vi "A-Lockin_Vsg-JKISM.vi"(8 "error in (no error)":errorcluster, 11 "SweepControl":refnum<class "SweepControl.lvclass">) -> (0 "error out":errorcluster)   [LabVIEW 2016, in "Transport.lvclass"]
uses:
  <userlib>/LevyLab/Transport/Transport/Transport.lvclass
  <userlib>/LevyLab/Lockin-Multichannel/Typedefs/AO-cluster.ctl
  <userlib>/LevyLab/Lockin-Multichannel/Typedefs/AO_Amp-array.ctl
  <userlib>/LevyLab/Lockin-Multichannel/Typedefs/AO_DC-array.ctl
  <userlib>/LevyLab/Lockin-Multichannel/Typedefs/AO_f-array.ctl
  <userlib>/LevyLab/Lockin-Multichannel/Typedefs/AO_phi-array.ctl
  <userlib>/LevyLab/Lockin-Multichannel/Typedefs/Function-array.ctl
  <userlib>/LevyLab/Lockin-Multichannel/Typedefs/Function-enum.ctl
  <userlib>/LevyLab/Transport/SweepControl/SweepControl.lvclass
  <userlib>/LevyLab/Transport/SweepControl/Typedefs/Cluster - ScanParamters.ctl
  <userlib>/LevyLab/Levylab Instruments/Instrument Types/Cryostat/Instrument.Cryostat.lvclass
  <userlib>/LevyLab/LV to ITX/LVtoITX.lvclass
  <userlib>/LevyLab/Transport/Control Experiment/Control Experiment.lvclass
panel:
  in  "OK":bool
  in  "Tab Control":enum32{"lockin/SG Control", "Data", "Other"}(tab)
  in  "Channels: AO":T1={"AO amp (V)"=[0.0002, 0.0, 0.0, 0.0, 0.0, 0.0, 0.0, 0.0], "AO DC (V)"=[0.00025, 0.0, 0.0, 0.0, 0.0, 0.0, 0.0, 0.0], "AO f (Hz)"=[13.0, 13.0, 13.0, 13.0, 13.0, 13.0, 13.0, 13.0], "AO phi (°)"=[0.0, 0.0, 0.0, 0.0, 0.0, 0.0, 0.0, 0.0], "function"=[enum."Sine", enum."Sine", enum."Sine", enum."Sine", enum."Sine", enum."Sine", enum."Sine", enum."Sine"], "I+"=[]} {"AO f (Hz)" min=0.001 max=10000.0; "AO DC (V)" format="%.3p"; "AO amp (V)" format="%.3p"}
  in  "Vmax (end)":dbl=1.0 format="%#_3p"
  in  "Vmin (start)":dbl format="%#_3p"
  in  "dV":dbl=0.1 format="%#_3p"
  in  "Experiment Description":string="write a description of THIS experiment here"
  in  "Experiment Folder":string="folder name"
  in  "wait after setting Vsg (ms)":u32
  in  "Initial wait (ms)":u32=100
  in  "side gate channel":i32=1 min=1
  in  "Physical Channel":tag="Dev2/ao0" caption="Back Gate Channel"
  in  "Sweep":enum16{"Vsg", "Vbg"}(ring)
  in  "cycles (1,2,...)":i32=1 min=1 step=1
  in  "phase":dbl
  in  "function (ramp)":enum16{"Ramp", "Triangle", "Sine"}(ring)
  in  "set parameter to initial value?":bool
  out "G 4T":cluster{"Y":dbl[], "Y":dbl[]}[](graph)
  out "Lockins":cluster{"Y":dbl[], "Y":dbl[]}[](graph)
  out "Lockins 2":cluster{"Y":dbl[], "Y":dbl[]}[](graph)
  # "1"
  # "2"
  # "3"
  # "4"
  # "5"
  # "6"
  # "7"
  # "8"
  # "dynamically name the traces"
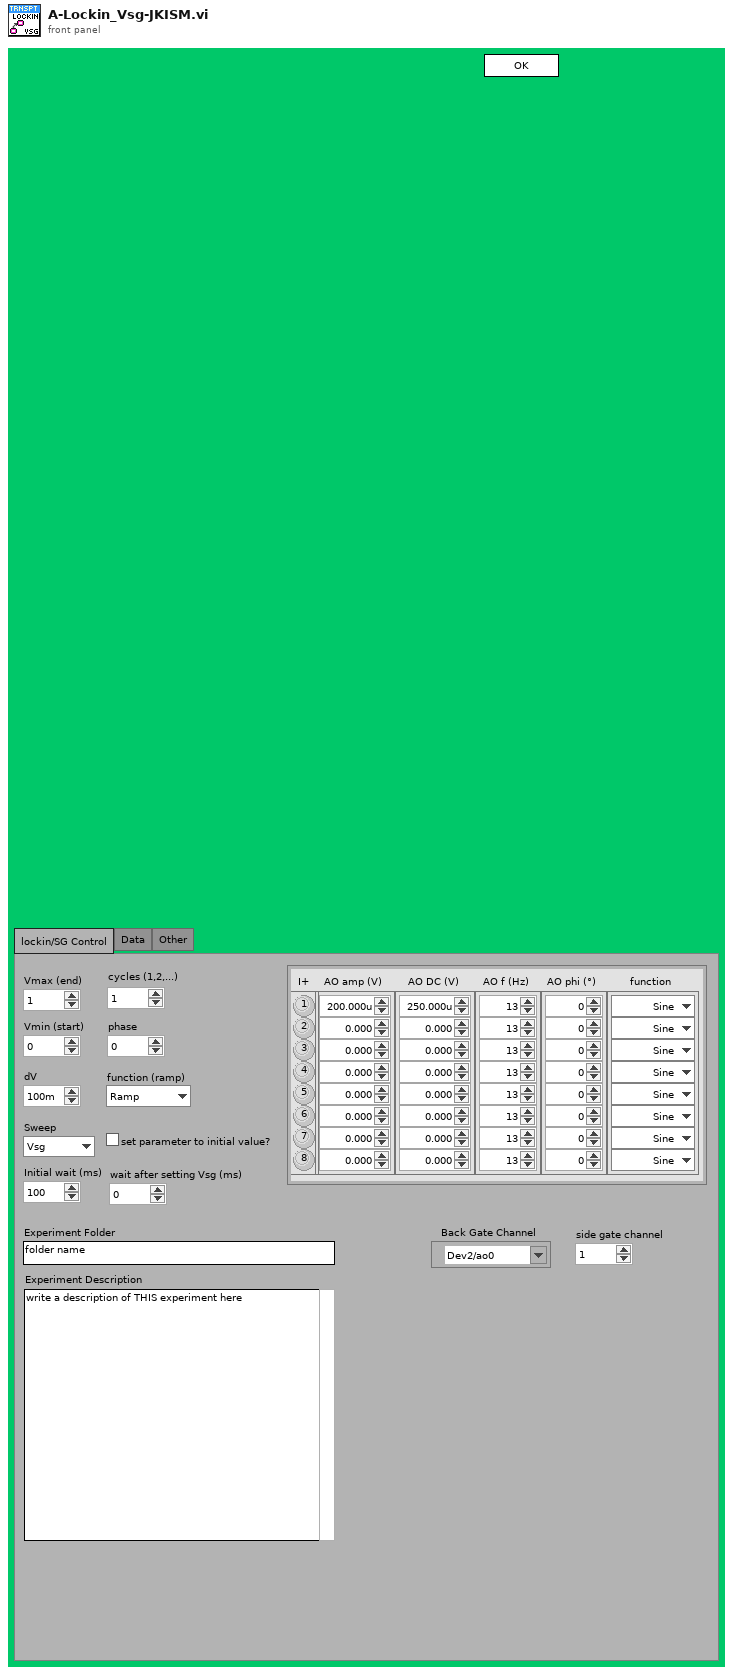
[diagram p1: front panel]
types:
  T1 = typedef "AO-cluster.ctl" = cluster{"AO amp (V)":T2, "AO DC (V)":T3, "AO f (Hz)":T4, "AO phi (°)":T5, "function":T6, "I+":bool[]}
  T2 = typedef "AO_Amp-array.ctl" = dbl[]
  T3 = typedef "AO_DC-array.ctl" = dbl[]
  T4 = typedef "AO_f-array.ctl" = dbl[]
  T5 = typedef "AO_phi-array.ctl" = dbl[]
  T6 = typedef "Function-array.ctl" = T7[]
  T7 = typedef "Function-enum.ctl" = enum16{"Sine", "Triangle", "Square", "Sawtooth"}
  T8 = enum32{"Bad", "Idle", "Run top level", "Running"}
  T9 = enum32{"invalid app kind", "Development System", "Run Time System", "Student Edition", "Embedded LabVIEW", "Evaluation", "Custom"}
  T10 = enum32{"Invalid", "Standard", "Closed", "Hidden", "Minimized", "Maximized"}
  T11 = typedef "SweepControl.lvclass/Cluster - ScanParamters.ctl" = cluster{"Start":dbl, "End":dbl, "Step":dbl, "Rate":dbl, "wait (ms)":u32, "Address":string, "Channel":i32}
  T12 = cluster{"Core":cluster{"Current VI Reference":refnum<vi>, "Close Panel on Exit?":bool}, "top level?":bool, "SweepControl":refnum<class "SweepControl.lvclass">, "Instrument":cluster{"Temperature":refnum<class "Instrument.Cryostat.lvclass">, "Magnet":refnum<class "Instrument.Cryostat.lvclass">, "Rotator":refnum<class "Instrument.Cryostat.lvclass">, "Level":refnum<class "Instrument.Cryostat.lvclass">}, "file":cluster{"path":path, "Experiment Folder":string, "device":string, "Comments":string}, "data":cluster{"Result X":dbl[], "Result Y":dbl[], "Data":cluster{"Y  Array":dbl[]}[], "wavenames":string[], "All Result X":dbl[][], "All Result Y":dbl[][]}, "lockin address":string, "Channels: AO":T1, "Temperature (K)":dbl, "Field (T)":dbl, "ramp rate (T/min)":dbl, "inner scan":T11, "All Parameters":dbl[], "loop index":i32, "Current Parameter":dbl}
  T13 = cluster{"Temperature":refnum<class "Instrument.Cryostat.lvclass">, "Magnet":refnum<class "Instrument.Cryostat.lvclass">, "Rotator":refnum<class "Instrument.Cryostat.lvclass">, "Level":refnum<class "Instrument.Cryostat.lvclass">}
  T14 = cluster{"Result X":dbl[], "Result Y":dbl[], "Data":cluster{"Y  Array":dbl[]}[], "wavenames":string[], "All Result X":dbl[][], "All Result Y":dbl[][]}
  T15 = cluster{"path":path, "Experiment Folder":string, "device":string, "Comments":string}
  T16 = cluster{"Current VI Reference":refnum<vi>, "Close Panel on Exit?":bool}
  T17 = typedef "SweepControl.lvclass/ScanParamters.ctl" = T11[]
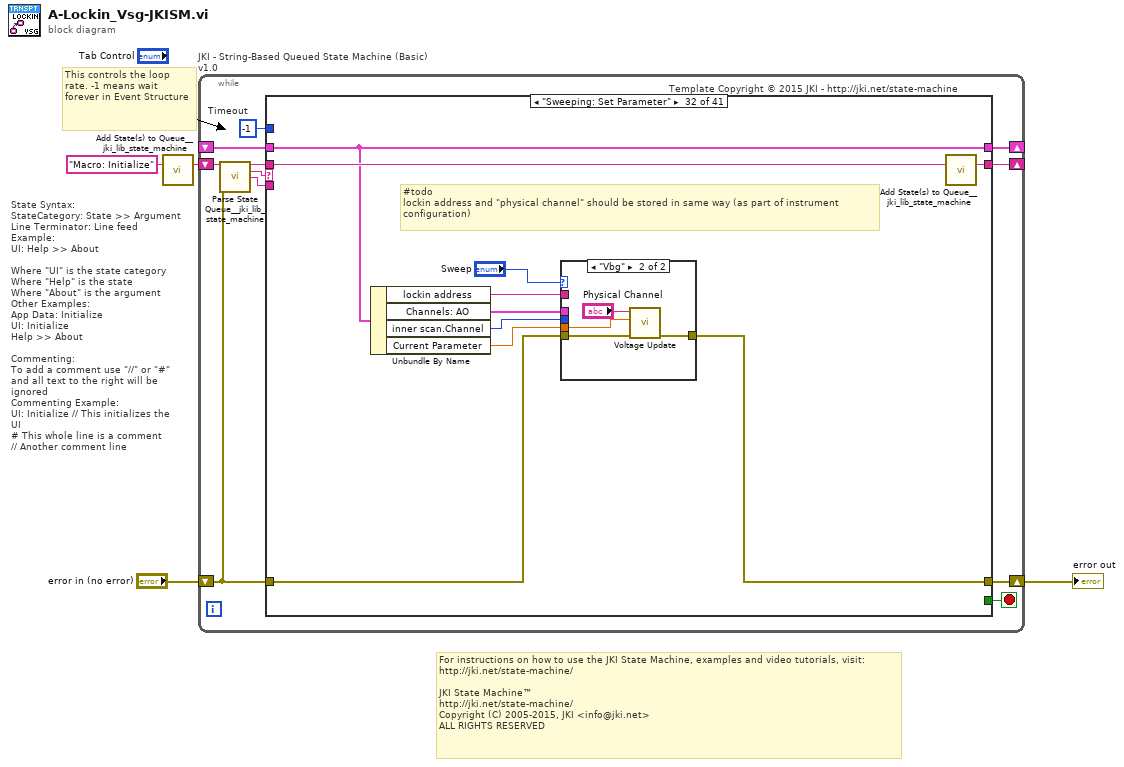
[diagram p0: block diagram]
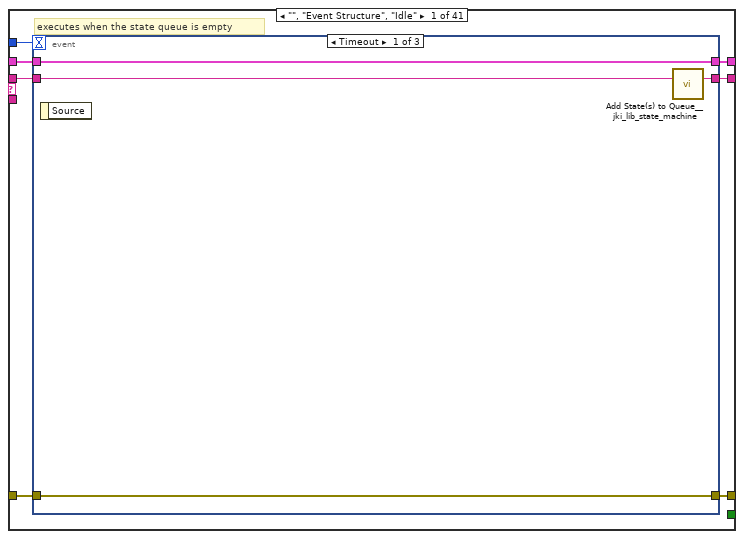
[diagram p2: hidden frame]
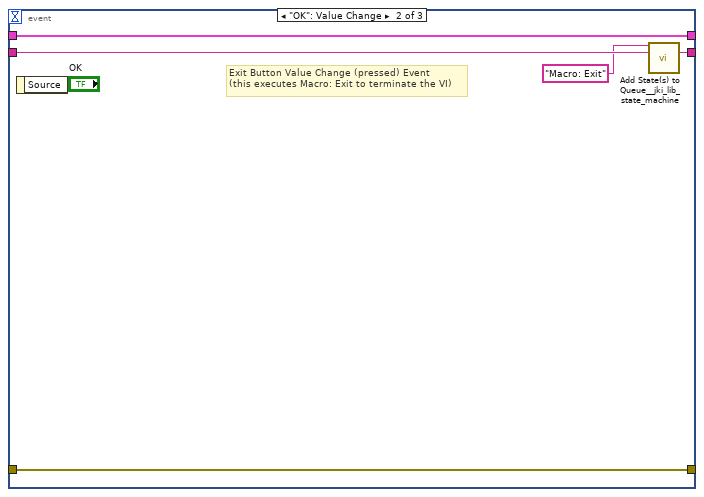
[diagram p3: hidden frame]
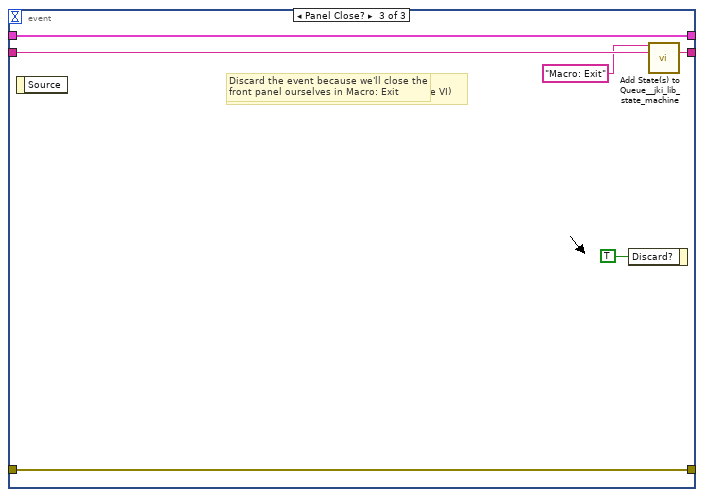
[diagram p4: hidden frame]
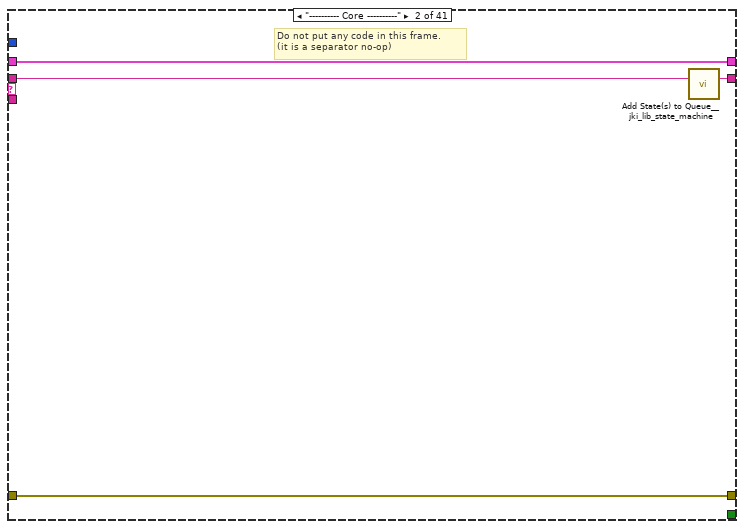
[diagram p5: hidden frame]
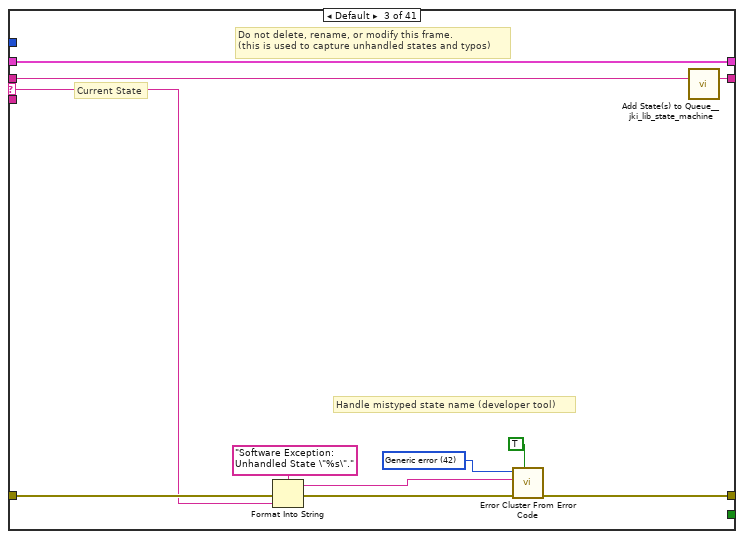
[diagram p6: hidden frame]
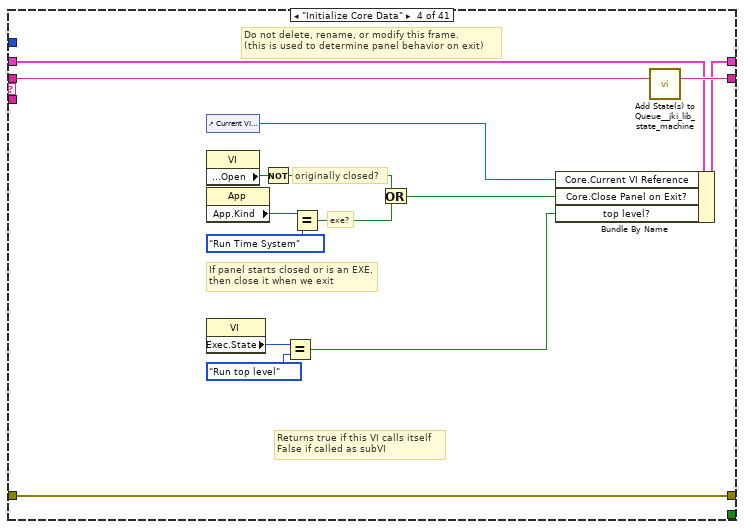
[diagram p7: hidden frame]
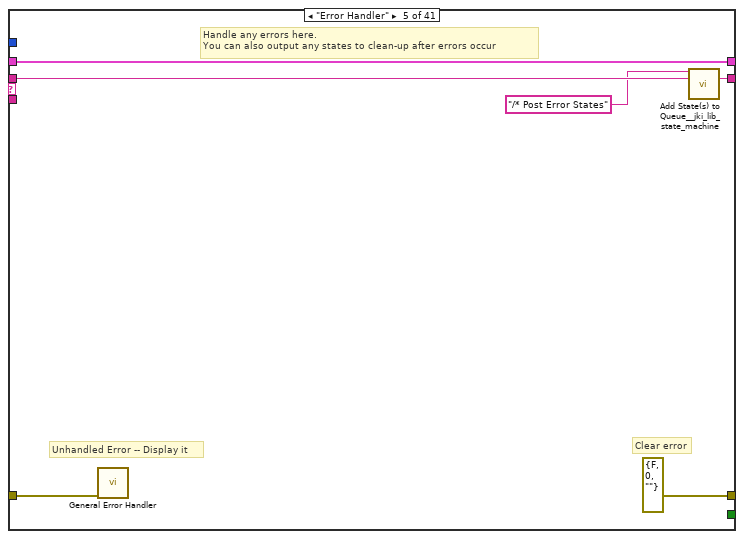
[diagram p8: hidden frame]
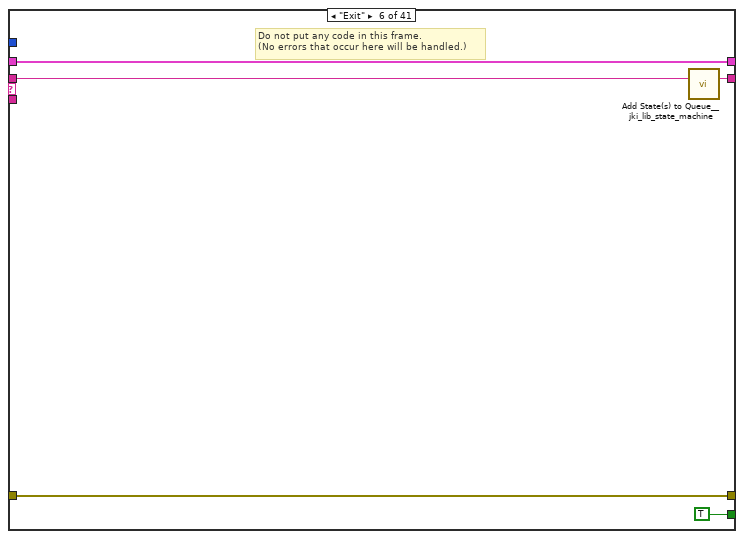
[diagram p9: hidden frame]
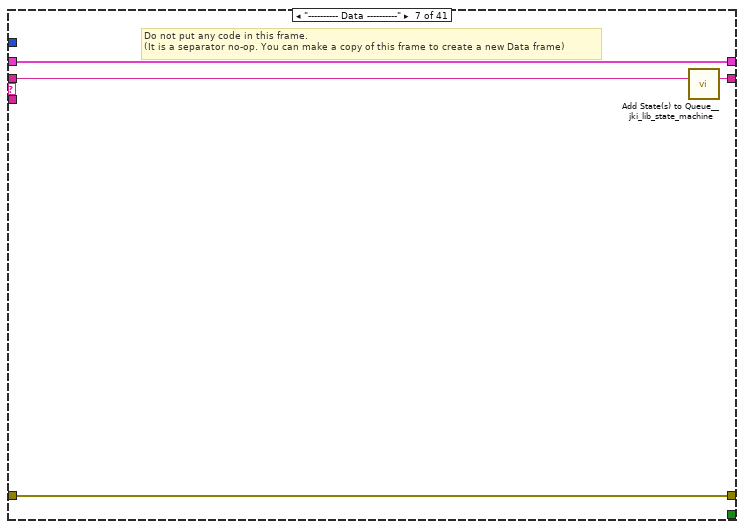
[diagram p10: hidden frame]
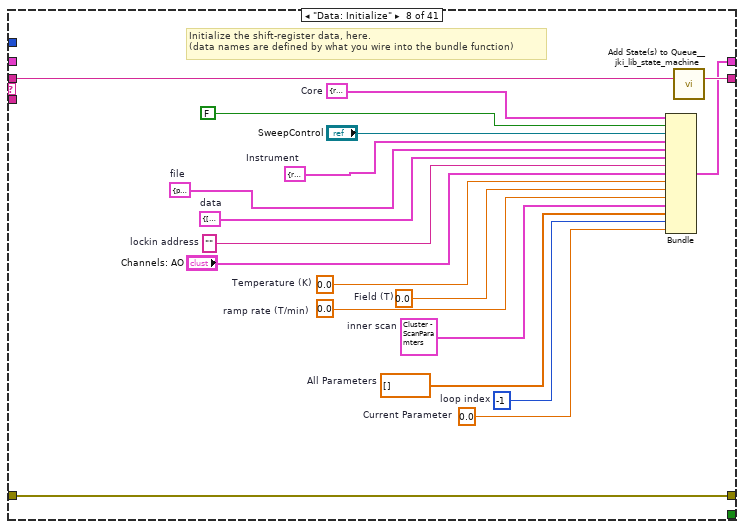
[diagram p11: hidden frame]
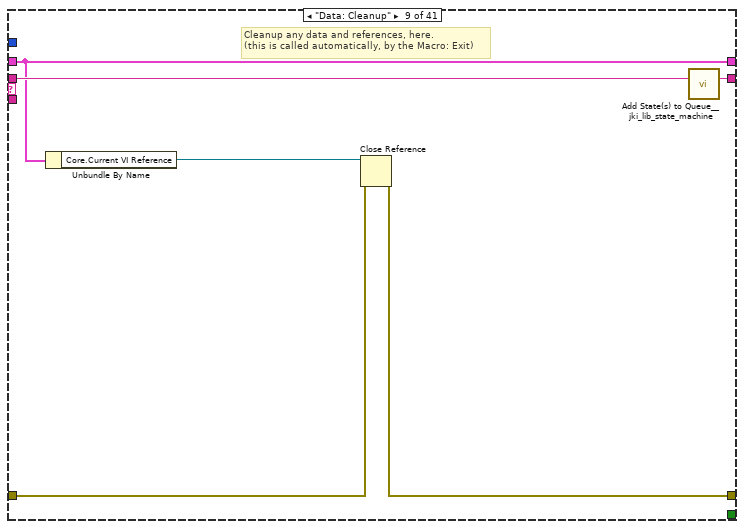
[diagram p12: hidden frame]
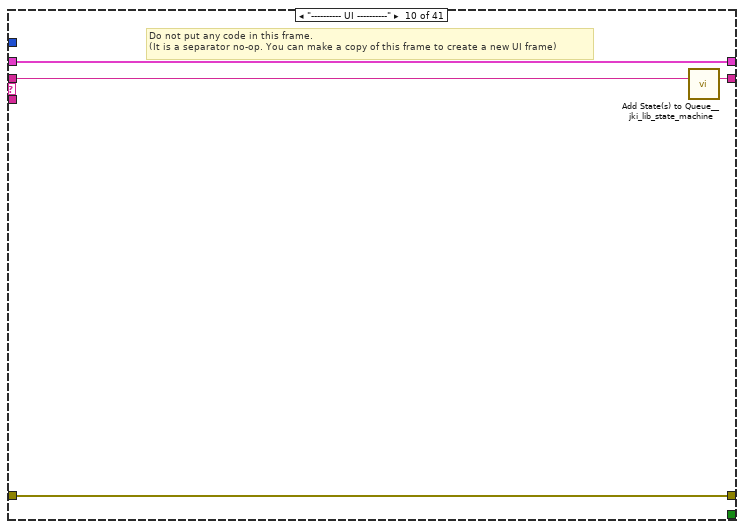
[diagram p13: hidden frame]
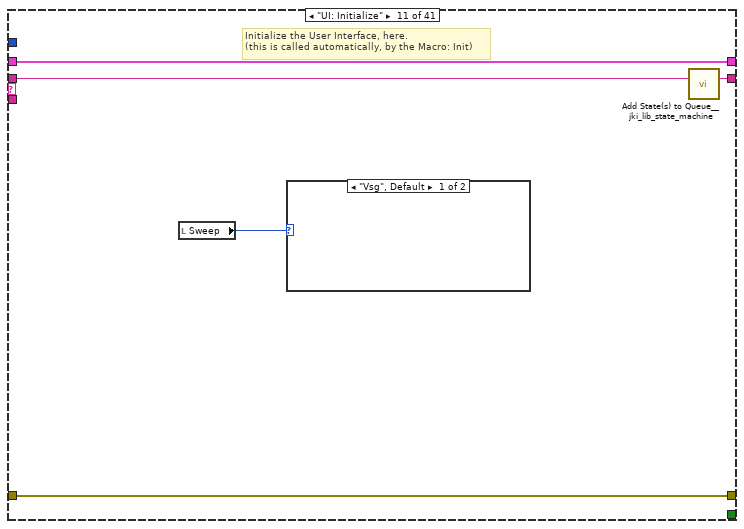
[diagram p14: hidden frame]
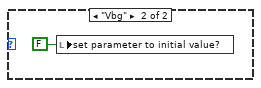
[diagram p15: hidden frame]
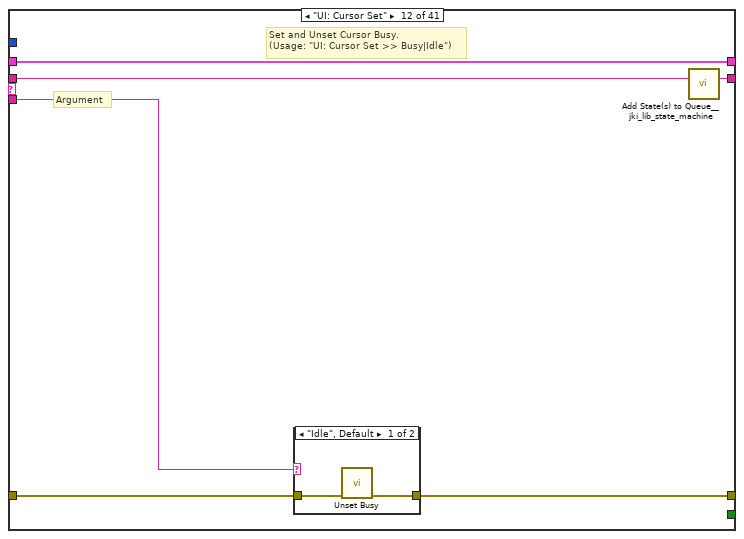
[diagram p16: hidden frame]
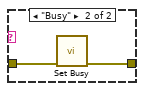
[diagram p17: hidden frame]
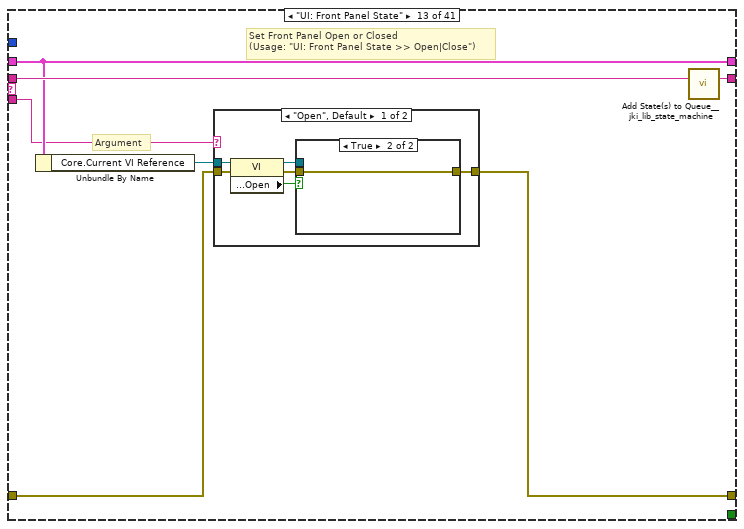
[diagram p18: hidden frame]
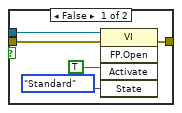
[diagram p19: hidden frame]
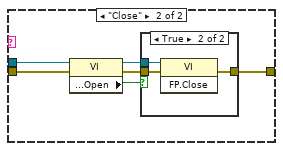
[diagram p20: hidden frame]
diagram:
  # "For instructions on how to use the JKI State Machine, examples and video tutorials, visit:\nhttp://jki.net/state-machine/\n\nJKI State Machine™\nhttp://jki.net/state-machine/\nCopyright (C) 2005-2015, JKI <info@jki.net>\nALL RIGHTS RESERVED"
  # "State Syntax:\nStateCategory: State >> Argument\nLine Terminator: Line feed\nExample:\nUI: Help >> About\n\nWhere \"UI\" is the state category\nWhere \"Help\" is the state\nWhere \"About\" is the argument\nOther Examples:\nApp Data: Initialize\nUI: Initialize\nHelp >> About\n\nCommenting:\nTo add a comment use \"//\" or \"#\" and all text to the right will be ignored\nCommenting Example:\nUI: Initialize // This initializes the UI\n# This whole line is a comment\n// Another comment line"
  # "This controls the loop rate. -1 means wait forever in Event Structure"
  n1 = call <vilib>:"Add State(s) to Queue__jki_lib_state_machine.vi"("State(s) in (\"\")"="Macro: Initialize") -> ("States Out"=w4:string)  [unwired: 14 in]
  n2 = while "JKI - String-Based Queued State Machine (Basic) v1.0" {
    shift-right: [w8] -> _
    shift-left: _ -> [w7]
    shift-right: [w11] -> w1
    shift-left: "error in (no error)" -> [w5]
    shift-right: [w10] -> _
    shift-left: w4 -> [w12]
    stop <- w9 stop-if-true
    w6 = -1  # Timeout
    # "Template Copyright © 2015 JKI - http://jki.net/state-machine"
    n3 = call <vilib>:"Parse State Queue__jki_lib_state_machine.vi"("State Queue"=w12, "Error In (no error)"=w5) -> ("Remaining States"=w14:string, "Current State"=w15:string, "Arguments"=w13:string)  [unwired: 11 in]
    n4 = case shown="\"Sweeping: Set Parameter\"" w15 {
      selector: w15 -> [_ _ w42 _ _ _ _ _ _ _ _ _ _ _ _ _ _ _ _ _ _ _ _ _ _ _ _ _ _ _ _ _ _ _ _ _ _ _ _ _ _]
      tunnel: w14 -> [w22 w41 w46 w67 w73 w78 w82 w101 w107 w111 w116 w123 w134 w160 w165 w170 w175 w180 w190 w194 w198 w202 w206 w212 w218 w222 w229 w260 w301 w305 w317 w341 w361 w367 w383 w399 w403 w420 w436 w449 w480]
      tunnel: w13 -> [_ _ _ _ _ _ _ _ _ _ _ w118 w128 _ _ _ _ _ _ _ _ _ _ _ _ _ _ _ _ _ _ _ _ _ _ _ _ _ _ _ _]
      tunnel: w7 -> [w20 w38 w44 w58 w70 w76 w79 _ w102 w108 w112 w121 w130 w157 w162 w167 w172 w177 w187 w191 w195 w199 w203 w209 w216 w219 w225 w254 w293 w302 w312 w339 w359 w362 w376 w391 w400 w417 w428 w438 w477]
      tunnel: [w19 w39 w48 w64 errorcluster {"status"=FALSE, "code"=0, "source"=""} ("error out") w75 w80 w98 w103 w109 w114 w119 w131 w158 w163 w168 w173 w178 w188 w192 w196 w200 w204 w210 w214 w220 w227 w256 w299 w303 w315 w333 w352 w364 w369 w397 w401 w418 w434 w447 w478] -> w11
      tunnel: w5 -> [w18 w39 w47 w64 w69 w75 w80 w98 w104 w109 w114 w120 w132 w158 w163 w168 w173 w178 w188 w192 w196 w200 w204 w210 w214 w220 w226 w257 w299 w303 w315 w335 w353 w365 w370 w397 w401 w418 w434 w447 w478]
      tunnel: [w21 w40 w45 w66 w72 w77 w81 w100 w106 w110 w115 w122 w133 w159 w164 w169 w174 w179 w189 w193 w197 w201 w205 w211 w217 w221 w228 w259 w300 w304 w316 w340 w360 w366 w382 w398 w402 w419 w435 w448 w479] -> w10
      tunnel: [_ _ _ _ _ TRUE _ _ _ _ _ _ _ _ _ _ _ _ _ _ _ _ _ _ _ _ _ _ _ _ _ _ _ _ _ _ _ _ _ _ _] -> w9
      tunnel: [w17 w38 w44 w65 w70 w76 w79 w99 w102 w108 w112 w121 w130 w157 w162 w167 w172 w177 w187 w191 w195 w199 w203 w208 w215 w219 w224 w258 w292 w302 w314 w339 w359 w362 w375 w391 w400 w416 w429 w437 w477] -> w8
      tunnel: w6 -> [w16 _ _ _ _ _ _ _ _ _ _ _ _ _ _ _ _ _ _ _ _ _ _ _ _ _ _ _ _ _ _ _ _ _ _ _ _ _ _ _ _]
      frame "", "Event Structure", "Idle" {
        # "executes when the state queue is empty"
        n5 = event shown="[0] Timeout" {
          selector: _ -> [_ _ _]
          dyn-events: _ -> [_ _ _]
          timeout: w16 -> [_ _ _]
          tunnel: w22 -> [w26 w31 w37]
          tunnel: [w25 w30 w36] -> w21
          tunnel: w20 -> [w23 w28 w34]
          tunnel: [w24 w29 w35] -> w19
          tunnel: w18 -> [w24 w29 w35]
          tunnel: [w23 w28 w34] -> w17
          event Timeout {
            n6 = event-data() -> ()  [unwired: 1 in, 1 out]
            n7 = call <vilib>:"Add State(s) to Queue__jki_lib_state_machine.vi"("State(s) in (\"\")"=w26) -> ("States Out"=w25:string)  [unwired: 14 in]
          }
          event "OK": Value Change {
            # "Exit Button Value Change (pressed) Event\n(this executes Macro: Exit to terminate the VI)"
            n8 = event-data() -> ()  [unwired: 1 in, 1 out]
            n9 = call <vilib>:"Add State(s) to Queue__jki_lib_state_machine.vi"("State(s) in Front (\"\")"="Macro: Exit", "State(s) in (\"\")"=w31) -> ("States Out"=w30:string)  [unwired: 13 in]
          }
          event Panel Close? {
            # "Discard the event because we'll close the front panel ourselves in Macro: Exit"
            # "Close Panel button (pressed) Event\n(this executes Macro: Exit to terminate the VI)"
            n10 = event-data() -> ()  [unwired: 1 in, 1 out]
            n11 = event-data("Discard?"=TRUE) -> ()  [unwired: 1 in, 1 out]
            n12 = call <vilib>:"Add State(s) to Queue__jki_lib_state_machine.vi"("State(s) in Front (\"\")"="Macro: Exit", "State(s) in (\"\")"=w37) -> ("States Out"=w36:string)  [unwired: 13 in]
          }
        }
      }
      frame "---------- Core ----------" {
        # "Do not put any code in this frame.\n(it is a separator no-op)"
        n13 = call <vilib>:"Add State(s) to Queue__jki_lib_state_machine.vi"("State(s) in (\"\")"=w41) -> ("States Out"=w40:string)  [unwired: 14 in]
      }
      frame Default {
        w51 = 42 items=["No error", "Argument error", "Memory is full", "Out of zone", "End of file", "File already open", "Generic file I/O error", "File not found", "File permission error", "Disk is full", "Duplicate path", "Too many files open", "System feature not enabled", "Resource file not found", "Cannot add resource", "Resource not found", "Image not found", "Image memory error", "Pen does not exist", "Config type invalid", "Config token not found", "Config parse error", "Config memory error", "Bad external code format", "Bad external code offset", "External code not present", "Null window", "Destroy window error", "Null menu", "Print aborted", "Bad print record", "Print driver error", "Windows error during printing", "Memory error during printing", "Print dialog error", "Generic print error", "Invalid device refnum", "Device not found", "Device parameter error", "Device unit error", "Cannot open device", "Device call aborted", "Generic error", "Cancelled by user", "Object ID too low", "Object ID too high", "Object not in heap", "Unknown heap", "Unknown object (invalid DefProc)", "Unknown object (DefProc not in table)", "Message out of range", "Invalid (null) method", "Unknown message", "Manager call not supported", "Bad address", "Network operation in progress", "Network operation timed out", "Connection is busy", "Network attribute not supported", "Network error", "Address in use", "System out of memory", "Connection aborted", "Connection refused", "Not connected", "Already connected", "Connection closed", "Initialization error (interapplication manager)", "Bad occurrence", "Wait on unbound occurrence handler", "Occurrence queue overflow", "Datalog type conflict", "Unused", "Unrecognized type (interapplication manager)", "Memory corrupt", "Failed to make temporary DLL", "Old CIN version", "Drag socket not found", "Failed to load drop-object", "Failed to register OLE object", "Failed to release OLE object", "Format specifier type mismatch", "Unknown format specifier", "Too few format specifiers", "Too many format specifiers", "Scan failed", "Newer CIN version", "Error converting to variant", "Runtime menu error", "Password tampered", "Variant attribute not found", "Incompatible variant data type", "Event data is not available", "Event Store is not present", "Occurrence is not found", "Event Queue is not created", "Event info is not available", "Refnum passed is NULL", "Error retrieving Class GUID", "Error retrieving CoClass GUID", "Error retrieving TypeLib GUID.", "Bad built application magic bytes.", "Specific driver is different from the specific driver associated with the Logical Name.", "There is no session opened to the class driver.", "Max Error", "MAX - Error with config objects", "MAX - Error loading configuration", "MAX - Group not supported"]
        # "Current State"
        # "Do not delete, rename, or modify this frame.\n(this is used to capture unhandled states and typos)"
        # "Handle mistyped state name (developer tool)"
        n14 = Format Into String(format string="Software Exception: Unhandled State \"%s\"." ("message"), error in=w47, w42) -> (resulting string=w50:string, error out=w49:errorcluster)  [unwired: 1 in]
        n15 = call <vilib>:"Error Cluster From Error Code.vi"("show call chain? (False)"=TRUE, "error in (no error)"=w49, "error message (\"\")"=w50, "error code (0)"=w51) -> ("error out"=w48:errorcluster)  [unwired: 5 in]
        n16 = call <vilib>:"Add State(s) to Queue__jki_lib_state_machine.vi"("State(s) in (\"\")"=w46) -> ("States Out"=w45:string)  [unwired: 14 in]
      }
      frame "Initialize Core Data" {
        # "Returns true if this VI calls itself\nFalse if called as subVI"
        # "Do not delete, rename, or modify this frame.\n(this is used to determine panel behavior on exit)"
        # "originally closed?"
        # "exe?"
        # "If panel starts closed or is an EXE, then close it when we exit"
        n17 = control-ref of="Current VI Reference"() -> (w56:refnum<vi>)
        n18 = property class="VI"() -> ("Front Panel.Open"=w63:bool)  [unwired: 2 in, 2 out]
        n19 = property class="App"() -> ("App.Kind"=w62:T9)  [unwired: 2 in, 2 out]
        n20 = property class="VI"() -> ("Exec.State"=w54:T8)  [unwired: 2 in, 2 out]
        n21 = Not(x=w63) -> (.not. x?=w60:bool)
        n22 = Equal?(x=w54, y=T8."Run top level" ("Execution:State")) -> (x = y?=w53:bool)
        n23 = Equal?(x=w62, y=T9."Run Time System" ("Application:Kind")) -> (x = y?=w59:bool)
        n24 = Or(x=w60, y=w59) -> (x .or. y?=w57:bool)
        n25 = Bundle By Name(cluster=w58, "Core.Current VI Reference"=w56, "Core.Close Panel on Exit?"=w57, "top level?"=w53) -> (w65:T12)
        n26 = call <vilib>:"Add State(s) to Queue__jki_lib_state_machine.vi"("State(s) in (\"\")"=w67) -> ("States Out"=w66:string)  [unwired: 14 in]
      }
      frame "Error Handler" {
        # "Unhandled Error -- Display it"
        # "Handle any errors here.\nYou can also output any states to clean-up after errors occur"
        # "Clear error"
        n27 = call <vilib>:"General Error Handler.vi"("error in (no error)"=w69) -> ()  [unwired: 10 in, 5 out]
        n28 = call <vilib>:"Add State(s) to Queue__jki_lib_state_machine.vi"("State(s) in Front (\"\")"="/* Post Error States", "State(s) in (\"\")"=w73) -> ("States Out"=w72:string)  [unwired: 13 in]
      }
      frame "Exit" {
        # "Do not put any code in this frame.\n(No errors that occur here will be handled.)"
        n29 = call <vilib>:"Add State(s) to Queue__jki_lib_state_machine.vi"("State(s) in (\"\")"=w78) -> ("States Out"=w77:string)  [unwired: 14 in]
      }
      frame "---------- Data ----------" {
        # "Do not put any code in this frame.\n(It is a separator no-op. You can make a copy of this frame to create a new Data frame)"
        n30 = call <vilib>:"Add State(s) to Queue__jki_lib_state_machine.vi"("State(s) in (\"\")"=w82) -> ("States Out"=w81:string)  [unwired: 14 in]
      }
      frame "Data: Initialize" {
        w83 = T13 {"Temperature"=refnum, "Magnet"=refnum, "Rotator"=refnum, "Level"=refnum}  # Instrument
        w86 = T14 {"Result X"=[], "Result Y"=[], "Data"=[], "wavenames"=[], "All Result X"=[], "All Result Y"=[]}  # data
        w84 = T15 {"path"=path "", "Experiment Folder"="", "device"="", "Comments"=""}  # file
        w88 = ""  # lockin address
        w89 = 0.0  # Current Parameter
        w90 = -1  # loop index
        w91 = 0.0  # ramp rate (T/min)
        w92 = dbl[] []  # All Parameters
        w93 = T11 {"Start"=0.14, "End"=-0.060000000000000005, "Step"=-0.060000000000000005, "Rate"=2.0, "wait (ms)"=10000, "Address"="Dev2/ao0", "Channel"=2}  # inner scan
        w94 = 0.0  # Field (T)
        w95 = 0.0  # Temperature (K)
        w97 = T16 {"Current VI Reference"=refnum, "Close Panel on Exit?"=FALSE}  # Core
        # "Initialize the shift-register data, here.\n(data names are defined by what you wire into the bundle function)"
        n31 = Bundle("Core"=w97, "top level?"=FALSE, "SweepControl"="SweepControl", "Instrument"=w83, "file"=w84, "data"=w86, "lockin address"=w88, "Channels: AO"="Channels: AO", "Temperature (K)"=w95, "Field (T)"=w94, "ramp rate (T/min)"=w91, "inner scan"=w93, "All Parameters"=w92, "loop index"=w90, "Current Parameter"=w89) -> (w99:T12)  [unwired: 1 in]
        n32 = call <vilib>:"Add State(s) to Queue__jki_lib_state_machine.vi"("State(s) in (\"\")"=w101) -> ("States Out"=w100:string)  [unwired: 14 in]
      }
      frame "Data: Cleanup" {
        # "Cleanup any data and references, here.\n(this is called automatically, by the Macro: Exit)"
        n33 = Unbundle By Name(w102) -> ("Core.Current VI Reference"=w105:refnum<vi>)
        n34 = Close Reference(reference=w105, error in (no error)=w104) -> (error out=w103:errorcluster)
        n35 = call <vilib>:"Add State(s) to Queue__jki_lib_state_machine.vi"("State(s) in (\"\")"=w107) -> ("States Out"=w106:string)  [unwired: 14 in]
      }
      frame "---------- UI ----------" {
        # "Do not put any code in this frame.\n(It is a separator no-op. You can make a copy of this frame to create a new UI frame)"
        n36 = call <vilib>:"Add State(s) to Queue__jki_lib_state_machine.vi"("State(s) in (\"\")"=w111) -> ("States Out"=w110:string)  [unwired: 14 in]
      }
      frame "UI: Initialize" {
        # "Initialize the User Interface, here.\n(this is called automatically, by the Macro: Init)"
        n37 = local read "Sweep"() -> (w113:enum16{"Vsg", "Vbg"})
        n38 = case shown="\"Vsg\", Default" w113 {
          frame "Vsg", Default {
          }
          frame "Vbg" {
            n39 = local write "set parameter to initial value?"(FALSE ("set parameter to initial value?")) -> ()
          }
        }
        n40 = call <vilib>:"Add State(s) to Queue__jki_lib_state_machine.vi"("State(s) in (\"\")"=w116) -> ("States Out"=w115:string)  [unwired: 14 in]
      }
      frame "UI: Cursor Set" {
        # "Argument"
        # "Set and Unset Cursor Busy.\n(Usage: \"UI: Cursor Set >> Busy|Idle\")"
        n41 = case shown="\"Idle\", Default" w118 {
          tunnel: w120 -> [w125 w127]
          tunnel: [w124 w126] -> w119
          frame "Idle", Default {
            n42 = call <vilib>:"Unset Busy.vi"("error in (no error)"=w125) -> ("error out"=w124:errorcluster)  [unwired: 10 in]
          }
          frame "Busy" {
            n43 = call <vilib>:"Set Busy.vi"("error in (no error)"=w127) -> ("error out"=w126:errorcluster)  [unwired: 9 in, 1 out]
          }
        }
        n44 = call <vilib>:"Add State(s) to Queue__jki_lib_state_machine.vi"("State(s) in (\"\")"=w123) -> ("States Out"=w122:string)  [unwired: 14 in]
      }
      frame "UI: Front Panel State" {
        # "Argument"
        # "Set Front Panel Open or Closed\n(Usage: \"UI: Front Panel State >> Open|Close\")"
        n45 = Unbundle By Name(w130) -> ("Core.Current VI Reference"=w129:refnum<vi>)
        n46 = case shown="\"Open\", Default" w128 {
          tunnel: w132 -> [w138 w151]
          tunnel: [w140 w152] -> w131
          tunnel: w129 -> [w139 w149]
          frame "Open", Default {
            n47 = property class="VI"(reference=w139, error in=w138) -> (reference out=w136:refnum<vi>, error out=w137:errorcluster, "Front Panel.Open"=w135:bool)
            n48 = case shown="True" w135 {
              tunnel: [w143 w146] -> w140
              tunnel: w137 -> [w142 w146]
              tunnel: w136 -> [w141 _]
              frame False {
                n49 = invoke class="VI" method="FP.Open"(reference=w141, error in=w142, "Activate"=TRUE, "State"=T10."Standard") -> (error out=w143:errorcluster)  [unwired: 1 in, 4 out]
              }
              frame True {
              }
            }
          }
          frame "Close" {
            n50 = property class="VI"(reference=w149, error in=w151) -> (reference out=w148:refnum<vi>, error out=w150:errorcluster, "Front Panel.Open"=w147:bool)
            n51 = case shown="True" w147 {
              tunnel: [w153 w156] -> w152
              tunnel: w150 -> [w153 w155]
              tunnel: w148 -> [_ w154]
              frame False {
              }
              frame True {
                n52 = invoke class="VI" method="FP.Close"(reference=w154, error in=w155) -> (error out=w156:errorcluster)  [unwired: 1 in, 2 out]
              }
            }
          }
        }
        n53 = call <vilib>:"Add State(s) to Queue__jki_lib_state_machine.vi"("State(s) in (\"\")"=w134) -> ("States Out"=w133:string)  [unwired: 14 in]
      }
      frame "---------- Macro ----------" {
        # "Do not put any code in this frame.\n(It is a separator no-op. You can make a copy of this frame to create a new Macro frame)"
        n54 = call <vilib>:"Add State(s) to Queue__jki_lib_state_machine.vi"("State(s) in (\"\")"=w160) -> ("States Out"=w159:string)  [unwired: 14 in]
      }
      frame "Macro: Initialize" {
        w161 = "Data: Initialize\nInitialize Core Data\nUI: Initialize\nUI: Front Panel State >> Open\nMacro: Sweep"  # Data: Initialize Initialize Core Data UI: Initialize UI: Front Panel State >> Open Macro: Sweep
        # "Initialization Macro\n(This is called once, when the VI starts)"
        n55 = call <vilib>:"Add State(s) to Queue__jki_lib_state_machine.vi"("State(s) in Front (\"\")"=w161, "State(s) in (\"\")"=w165) -> ("States Out"=w164:string)  [unwired: 13 in]
      }
      frame "Macro: Sweep" {
        n56 = call <vilib>:"Add State(s) to Queue__jki_lib_state_machine.vi"("State(s) in Front (\"\")"="Sweep: Get\nSweep: Get Remote\nSweep: Define Sweep\nSweeping: Sweeping", "State(s) in (\"\")"=w170) -> ("States Out"=w169:string)  [unwired: 13 in]
      }
      frame "Macro: Sweeping" {
        n57 = call <vilib>:"Add State(s) to Queue__jki_lib_state_machine.vi"("State(s) in Front (\"\")"="Sweeping: Set Parameter\nSweeping: Wait\nSweeping: Wait New AI\nSweeping: Get Result\nSweeping: Plot", "State(s) in (\"\")"=w175) -> ("States Out"=w174:string)  [unwired: 13 in]
      }
      frame "Macro: Save" {
        n58 = call <vilib>:"Add State(s) to Queue__jki_lib_state_machine.vi"("State(s) in Front (\"\")"="File: Prepare 0D Data\nFile: Prepare 1D Data\nFile: Prepare 2D Data\nFile: Save ITX", "State(s) in (\"\")"=w180) -> ("States Out"=w179:string)  [unwired: 13 in]
      }
      frame "Macro: Exit" {
        # "Exit Macro\n(This is called once, when the VI exits)"
        n59 = Unbundle By Name(w187) -> ("Core.Close Panel on Exit?"=w186:bool)
        n60 = Select(t="UI: Front Panel State >> Close", s=w186, f="") -> (s? t:f=w183:string)
        n61 = call <vilib>:"Add State(s) to Queue__jki_lib_state_machine.vi"("State(s) in (\"\")"=w183, "State(s) at Back (\"\")"="Data: Cleanup\nExit") -> ("States Out"=w181:string)  [unwired: 13 in]
        n62 = call <vilib>:"Add State(s) to Queue__jki_lib_state_machine.vi"("State(s) in Front (\"\")"=w181, "State(s) in (\"\")"=w190) -> ("States Out"=w189:string)  [unwired: 13 in]
      }
      frame "---------- Lockin ----------" {
        # "Template Separator\n(You can make a copy of, or modify, this frame)"
        n63 = call <vilib>:"Add State(s) to Queue__jki_lib_state_machine.vi"("State(s) in (\"\")"=w194) -> ("States Out"=w193:string)  [unwired: 14 in]
      }
      frame "Lockin: 1" {
        # "Your code here.\n(You can make a copy of, or modify, this frame)"
        n64 = call <vilib>:"Add State(s) to Queue__jki_lib_state_machine.vi"("State(s) in (\"\")"=w198) -> ("States Out"=w197:string)  [unwired: 14 in]
      }
      frame "Lockin: 2" {
        # "Your code here.\n(You can make a copy of, or modify, this frame)"
        n65 = call <vilib>:"Add State(s) to Queue__jki_lib_state_machine.vi"("State(s) in (\"\")"=w202) -> ("States Out"=w201:string)  [unwired: 14 in]
      }
      frame "---------- Instrument ----------" {
        # "Template Separator\n(You can make a copy of, or modify, this frame)"
        n66 = call <vilib>:"Add State(s) to Queue__jki_lib_state_machine.vi"("State(s) in (\"\")"=w206) -> ("States Out"=w205:string)  [unwired: 14 in]
      }
      frame "Instrument: Get Temperature" {
        # "#todo add subVI to read temp"
        n67 = Unbundle By Name(w209) -> ()  [unwired: 1 out]
        n68 = Bundle By Name(cluster=w209, "Temperature (K)"=0.0) -> (w208:T12)
        n69 = call <vilib>:"Add State(s) to Queue__jki_lib_state_machine.vi"("State(s) in (\"\")"=w212) -> ("States Out"=w211:string)  [unwired: 14 in]
      }
      frame "Instrument: Get Magnet" {
        w213 = 0.0 ("ramp rate (T/min)")
        # "#todo add subVI to read B"
        n70 = Unbundle By Name(w216) -> ()  [unwired: 1 out]
        n71 = Bundle By Name(cluster=w216, "Field (T)"=w213, "ramp rate (T/min)"=w213) -> (w215:T12)
        n72 = call <vilib>:"Add State(s) to Queue__jki_lib_state_machine.vi"("State(s) in (\"\")"=w218) -> ("States Out"=w217:string)  [unwired: 14 in]
      }
      frame "---------- Sweep ----------" {
        # "Template Separator\n(You can make a copy of, or modify, this frame)"
        n73 = call <vilib>:"Add State(s) to Queue__jki_lib_state_machine.vi"("State(s) in (\"\")"=w222) -> ("States Out"=w221:string)  [unwired: 14 in]
      }
      frame "Sweep: Get" {
        n74 = Unbundle By Name(w225) -> ("top level?"=w223:bool)
        n75 = case shown="False" w223 {
          tunnel: [w239 w249] -> w227
          tunnel: w226 -> [w233 w250]
          tunnel: w225 -> [w232 w253]
          tunnel: [w231 w252] -> w224
          frame False {
            # "#todo\nThese need to be read from the FGV when\nthis is called as top level VI (do not get from the class\nwire)"
            n76 = Unbundle By Name(w232) -> ("SweepControl"=w244:refnum<class "SweepControl.lvclass">)
            n77 = call-dynamic "Read path.vi"("error in (no error)"=w233, "SweepControl in"=w244) -> ("error out"=w242:errorcluster, "path"=w241:path, "SweepControl out"=w243:refnum<class "SweepControl.lvclass">)  [unwired: 7 in]
            n78 = call-dynamic "Read device.vi"("error in (no error)"=w242, "SweepControl in"=w243) -> ("error out"=w238:errorcluster, "device"=w240:string, "SweepControl out"=w237:refnum<class "SweepControl.lvclass">)  [unwired: 7 in]
            n79 = call-dynamic "Read Comments.vi"("error in (no error)"=w238, "SweepControl in"=w237) -> ("error out"=w235:errorcluster, "Comments"=w234:string, "SweepControl out"=w236:refnum<class "SweepControl.lvclass">)  [unwired: 7 in]
            n80 = call-dynamic "Read Instrument.vi"("error in (no error)"=w235, "SweepControl in"=w236) -> ("error out"=w239:errorcluster, "Instrument"=w230:T13)  [unwired: 7 in, 1 out]
            n81 = Bundle By Name(cluster=w232, "file.path"=w241, "file.device"=w240, "file.Comments"=w234, "Instrument"=w230) -> (w231:T12)
          }
          frame True {
            # "#todo\nThese need to be read from the FGV when\nthis is called as top level VI (do not get from the class\nwire)"
            # "TOP LEVEL VI"
            n82 = Unbundle By Name(w253) -> ("lockin address"=w251:string)
            n83 = call <userlib>:"Initialize Experiment.vi"("lockin address"=w251, "error in (no error)"=w250, "Experiment Comments"="Experiment Description") -> ("error out"=w249:errorcluster, "Comments"=w245:string, "device"=w247:string, "path"=w248:path)  [unwired: 5 in]
            n84 = Bundle By Name(cluster=w253, "file.path"=w248, "file.device"=w247, "file.Comments"=w245) -> (w252:T12)
          }
        }
        n85 = call <vilib>:"Add State(s) to Queue__jki_lib_state_machine.vi"("State(s) in (\"\")"=w229) -> ("States Out"=w228:string)  [unwired: 14 in]
      }
      frame "Sweep: Get Remote" {
        # "#todo\nexperiment folder name should be generated automatically\n(### - Calling VI - Something Descriptive)"
        n86 = Unbundle By Name(w254) -> ("top level?"=w255:bool)
        n87 = case shown="True" w255 {
          tunnel: w254 -> [w277 w282]
          tunnel: [w276 w283] -> w258
          tunnel: w257 -> [w279 w281]
          tunnel: [w266 w281] -> w256
          frame False {
            n88 = Unbundle By Name(w277) -> ("SweepControl"=w275:refnum<class "SweepControl.lvclass">)
            n89 = call-dynamic "Read Channels_ AO.vi"("error in (no error)"=w279, "SweepControl in"=w275) -> ("error out"=w265:errorcluster, "Channels: AO"=w263:T1, "SweepControl out"=w264:refnum<class "SweepControl.lvclass">)  [unwired: 7 in]
            n90 = call-dynamic "Read Experiment folder name.vi"("error in (no error)"=w265, "SweepControl in"=w264) -> ("error out"=w272:errorcluster, "Experiment folder name"=w278:string, "SweepControl out"=w271:refnum<class "SweepControl.lvclass">)  [unwired: 7 in]
            n91 = call-dynamic "Read Sorted scan parameters.vi"("error in (no error)"=w272, "SweepControl in"=w271) -> ("error out"=w266:errorcluster, "Sorted scan parameters"=w274:cluster{T17}[])  [unwired: 7 in, 1 out]
            n92 = Index Array(array=w274) -> (element=w273:cluster{T17})  [unwired: 1 in]
            n93 = Unbundle(w273) -> (w262:T17)
            n94 = Index Array(array=w262) -> (element=w261:T11)  [unwired: 1 in]
            n95 = Unbundle By Name(w261) -> ("Start"=w270:dbl, "End"=w269:dbl, "Step"=w268:dbl, "Channel"=w267:i32)
            n96 = Bundle By Name(cluster=w277, "Channels: AO"=w263, "file.Experiment Folder"=w278, "inner scan"=w261) -> (w276:T12)
            n97 = local write "Vmax (end)"(w269) -> ()
            n98 = local write "side gate channel"(w267) -> ()
            n99 = local write "Vmin (start)"(w270) -> ()
            n100 = local write "dV"(w268) -> ()
          }
          frame True {
            n101 = Bundle By Name(cluster=w282, "file.Experiment Folder"="Experiment Folder", "inner scan.Start"="Vmin (start)", "inner scan.End"="Vmax (end)", "inner scan.Step"="dV", "inner scan.Channel"="side gate channel") -> (w283:T12)
          }
        }
        n102 = call <vilib>:"Add State(s) to Queue__jki_lib_state_machine.vi"("State(s) in (\"\")"=w260) -> ("States Out"=w259:string)  [unwired: 14 in]
      }
      frame "Sweep: Define Sweep" {
        n103 = Unbundle By Name(w293) -> ("inner scan.End"=w296:dbl, "inner scan.Start"=w295:dbl, "inner scan.Step"=w294:dbl)
        n104 = call <userlib>:"Max_Min_conversion.vi"("Min"=w295, "Max"=w296) -> ("offset"=w298:dbl, "Amplitude"=w297:dbl)  [unwired: 8 in]
        n105 = call <userlib>:"Ramp.vi"("phase"="phase", "function (ramp)"="function (ramp)", "cycles (1,2,...)"="cycles (1,2,...)", "step size"=w294, "offset"=w298, "amplitude"=w297) -> ("Waveform Graph"=w291:dbl[])  [unwired: 3 in, 2 out]
        n106 = Bundle By Name(cluster=w293, "All Parameters"=w291) -> (w292:T12)
        n107 = call <vilib>:"Add State(s) to Queue__jki_lib_state_machine.vi"("State(s) in (\"\")"=w301) -> ("States Out"=w300:string)  [unwired: 14 in]
      }
      frame "---------- Sweeping ----------" {
        # "Template Separator\n(You can make a copy of, or modify, this frame)"
        n108 = call <vilib>:"Add State(s) to Queue__jki_lib_state_machine.vi"("State(s) in (\"\")"=w305) -> ("States Out"=w304:string)  [unwired: 14 in]
      }
      frame "Sweeping: Sweeping" {
        n109 = Unbundle By Name(w312) -> ("All Parameters"=w309:dbl[], "loop index"=w308:i32)
        n110 = Array Size(array=w309) -> (size(s)=w311:i32)
        n111 = Greater?(x=w311, y=w308) -> (0:w307:bool)
        n112 = case shown="False" w307 {
          tunnel: [w322 -1] -> w313
          tunnel: [w321 w329] -> w310
          tunnel: w309 -> [w320 w330]
          tunnel: w308 -> [w319 _]
          tunnel: ["Macro: Sweeping\nSweeping: Sweeping" w323] -> w306
          frame True {
            n113 = Index Array(array=w320, index=w319) -> (element=w321:dbl)
            n114 = Increment(x=w319) -> (x+1=w322:i32)
          }
          frame False {
            n115 = Index Array(array=w330) -> (element=w329:dbl)  [unwired: 1 in]
            n116 = Select(t="Sweeping: Set Parameter", s="set parameter to initial value?", f="") -> (s? t:f=w324:string)
            n117 = call <vilib>:"Add State(s) to Queue__jki_lib_state_machine.vi"("State(s) in Front (\"\")"=w324, "State(s) at Back (\"\")"="Macro: Save\nMacro: Exit") -> ("States Out"=w323:string)  [unwired: 13 in]
          }
        }
        n118 = Bundle By Name(cluster=w312, "loop index"=w313, "Current Parameter"=w310) -> (w314:T12)
        n119 = call <vilib>:"Add State(s) to Queue__jki_lib_state_machine.vi"("State(s) in Front (\"\")"=w306, "State(s) in (\"\")"=w317) -> ("States Out"=w316:string)  [unwired: 13 in]
      }
      frame "Sweeping: Set Parameter" {
        # "#todo\nlockin address and \"physical channel\" should be stored in same way (as part of instrument\nconfiguration)"
        n120 = Unbundle By Name(w339) -> ("lockin address"=w332:string, "Channels: AO"=w338:T1, "inner scan.Channel"=w337:i32, "Current Parameter"=w336:dbl)
        n121 = case shown="\"Vbg\"" "Sweep" {
          tunnel: w338 -> [w347 _]
          tunnel: w337 -> [w346 _]
          tunnel: w336 -> [w345 w350]
          tunnel: [w344 w348] -> w333
          tunnel: w335 -> [w343 w349]
          tunnel: w332 -> [w342 _]
          frame "Vsg", Default {
            n122 = call <userlib>:"configAO_DC.vi"("address"=w342, "error in (no error)"=w343, "new DC (V)"=w345, "AO Channel"=w346, "Channels: AO"=w347) -> ("error out"=w344:errorcluster)  [unwired: 5 in, 1 out]
          }
          frame "Vbg" {
            n123 = call <vilib>:"Voltage Update.vi"("error in (no error)"=w349, "Voltage Output"=w350, "Physical Channel"="Physical Channel") -> ("error out"=w348:errorcluster)  [unwired: 7 in, 1 out]
          }
        }
        n124 = call <vilib>:"Add State(s) to Queue__jki_lib_state_machine.vi"("State(s) in (\"\")"=w341) -> ("States Out"=w340:string)  [unwired: 14 in]
      }
      frame "Sweeping: Wait" {
        n125 = Unbundle By Name(w359) -> ("loop index"=w355:i32)
        n126 = Equal To 0?(x=w355) -> (x = 0?=w358:bool)
        n127 = Select(t="Initial wait (ms)", s=w358, f="wait after setting Vsg (ms)") -> (s? t:f=w354:u32)
        n128 = call <userlib>:"Wait (ms)__ogtk.vi"("error in (no error)"=w353, "milliseconds to wait"=w354) -> ("error out"=w352:errorcluster)  [unwired: 8 in, 1 out]
        n129 = call <vilib>:"Add State(s) to Queue__jki_lib_state_machine.vi"("State(s) in (\"\")"=w361) -> ("States Out"=w360:string)  [unwired: 14 in]
      }
      frame "Sweeping: Wait New AI" {
        n130 = Unbundle By Name(w362) -> ("lockin address"=w363:string)
        n131 = call <userlib>:"waitForNewWaveforms.vi"("address"=w363, "error in (no error)"=w365) -> ("error out"=w364:errorcluster)  [unwired: 8 in, 1 out]
        n132 = call <vilib>:"Add State(s) to Queue__jki_lib_state_machine.vi"("State(s) in (\"\")"=w367) -> ("States Out"=w366:string)  [unwired: 14 in]
      }
      frame "Sweeping: Get Result" {
        n133 = Unbundle By Name(w376) -> ("data.All Result X"=w378:dbl[][], "data.All Result Y"=w377:dbl[][], "lockin address"=w381:string)
        n134 = call <userlib>:"readResults.vi"("address"=w381, "error in (no error)"=w370) -> ("error out"=w369:errorcluster, "Results"=w368:dbl[][])  [unwired: 7 in, 1 out]
        n135 = Array Size(array=w368) -> (size(s)=w380:i32[])
        n136 = Index Array(array=w380) -> (element=w379:i32)  [unwired: 1 in]
        n137 = for {
          N: w379 -> [_]
          tunnel: w368 -> [w389]
          tunnel: [w387] -> w374 mode=indexing
          tunnel: [w386] -> w373 mode=indexing
          i -> [w388]
          w384 = 1  # y
          w385 = 0  # x
          # "extract x and y"
          n138 = Index Array(array=w389, index (row) #1=w388, index (col) #1=w385, index (row) #2=w388, index (col) #2=w384) -> (element #1=w387:dbl, element #2=w386:dbl)
        }
        n139 = Build Array (concatenate)(w378, w374) -> (w371:dbl[][])
        n140 = Build Array (concatenate)(w377, w373) -> (w372:dbl[][])
        n141 = Bundle By Name(cluster=w376, "data.All Result X"=w371, "data.Result X"=w374, "data.All Result Y"=w372, "data.Result Y"=w373) -> (w375:T12)
        n142 = call <vilib>:"Add State(s) to Queue__jki_lib_state_machine.vi"("State(s) in (\"\")"=w383) -> ("States Out"=w382:string)  [unwired: 14 in]
      }
      frame "Sweeping: Plot" {
        n143 = Unbundle By Name(w391) -> ("loop index"=w394:i32, "data.Result X"=w392:dbl[], "Current Parameter"=w390:dbl)
        n144 = Equal To 0?(x=w394) -> (x = 0?=w393:bool)
        n145 = call <userlib>:"LockinVsgGraphs.vi"("reset?"=w393, "parameter in"=w390, "X array in"=w392) -> ("R (ohms) vs Parameter Out 2"=→"Lockins" →"Lockins 2":cluster{"Y":dbl[], "Y":dbl[]}[], "G (e2/h) vs Parameter Out"=→"G 4T":cluster{"Y":dbl[], "Y":dbl[]}[])  [unwired: 5 in, 2 out]
        n146 = call <vilib>:"Add State(s) to Queue__jki_lib_state_machine.vi"("State(s) in (\"\")"=w399) -> ("States Out"=w398:string)  [unwired: 14 in]
      }
      frame "---------- File ----------" {
        # "Template Separator\n(You can make a copy of, or modify, this frame)"
        n147 = call <vilib>:"Add State(s) to Queue__jki_lib_state_machine.vi"("State(s) in (\"\")"=w403) -> ("States Out"=w402:string)  [unwired: 14 in]
      }
      frame "File: Prepare 0D Data" {
        # "#todo\nthese should be made dynamically from \"get/set parameter\""
        n148 = Unbundle By Name(w417) -> ("data.Data"=w415:cluster{"Y  Array":dbl[]}[], "data.wavenames"=w414:string[], "Temperature (K)"=w408:dbl, "Field (T)"=w407:dbl, "ramp rate (T/min)"=w406:dbl)
        n149 = Get Date/Time In Seconds() -> (seconds since 1Jan1904=w410:timestamp)
        n150 = To Double Precision Float(number=w410) -> (double precision float=w409:dbl)
        n151 = Build Array(w409, w408, w407, w406) -> (w404:dbl[])
        n152 = for {
          tunnel: [w422] -> w405 mode=concatenating
          tunnel: w404 -> [w421] mode=indexing
          # "build cluster array"
          n153 = Build Array(w421) -> (w423:dbl[])
          n154 = Build Cluster Array(w423) -> (w422:cluster{dbl[]}[])
        }
        n155 = Build Array (concatenate)(w415, w405) -> (w412:cluster{"Y  Array":dbl[]}[])
        n156 = Build Array (concatenate)(w414, string[] ["time", "T", "B", "B_rate"] ("wavenames (.Vx, etc)")) -> (w413:string[])
        n157 = Bundle By Name(cluster=w417, "data.Data"=w412, "data.wavenames"=w413) -> (w416:T12)
        n158 = call <vilib>:"Add State(s) to Queue__jki_lib_state_machine.vi"("State(s) in (\"\")"=w420) -> ("States Out"=w419:string)  [unwired: 14 in]
      }
      frame "File: Prepare 1D Data" {
        # "#todo\nthese should be made dynamically from \"get/set parameter\""
        # "Template Separator\n(You can make a copy of, or modify, this frame)"
        n159 = Unbundle By Name(w428) -> ("data.Data"=w433:cluster{"Y  Array":dbl[]}[], "data.wavenames"=w432:string[], "All Parameters"=w425:dbl[])
        n160 = Build Cluster Array(w425) -> (w424:cluster{"All Parameters":dbl[]}[])
        n161 = Build Array("Vsg" ("wavenames")) -> (w426:string[])
        n162 = Build Array (concatenate)(w433, w424) -> (w430:cluster{"All Parameters":dbl[]}[])
        n163 = Build Array (concatenate)(w432, w426) -> (w431:string[])
        n164 = Bundle By Name(cluster=w428, "data.Data"=w430, "data.wavenames"=w431) -> (w429:T12)
        n165 = call <vilib>:"Add State(s) to Queue__jki_lib_state_machine.vi"("State(s) in (\"\")"=w436) -> ("States Out"=w435:string)  [unwired: 14 in]
      }
      frame "File: Prepare 2D Data" {
        # "dynamically format lockin data cluster & wavenames\n--> less wires & cleaner code\n--> number of channels is scalable"
        n166 = Unbundle By Name(w438) -> ("data.Data"=w446:cluster{"Y  Array":dbl[]}[], "data.wavenames"=w445:string[], "data.All Result X"=w442:dbl[][], "data.All Result Y"=w441:dbl[][])
        n167 = flat-sequence {
          tunnel: w442 -> [w459]
          tunnel: w441 -> [w458]
          tunnel: [w451] -> w439
          tunnel: [w450] -> w440
          frame #0 {
            # "build cluster array(s) of multiple 1D data, dynamically name waves"
            n168 = Transpose 2D Array(2D array=w459) -> (transposed array=w457:dbl[][])
            n169 = Transpose 2D Array(2D array=w458) -> (transposed array=w456:dbl[][])
            n170 = for {
              tunnel: w457 -> [w469] mode=indexing
              tunnel: w456 -> [w468] mode=indexing
              tunnel: [w467] -> w455 mode=concatenating
              tunnel: [w466] -> w454 mode=concatenating
              tunnel: [w461] -> w453 mode=indexing
              tunnel: [w460] -> w452 mode=indexing
              i -> [w463]
              n171 = Number To Decimal String(number=w463) -> (decimal integer string=w462:string)  [unwired: 1 in]
              n172 = Concatenate Strings("X" ("wavenames"), w462) -> (w461:string)
              n173 = Concatenate Strings("Y" ("wavenames"), w462) -> (w460:string)
              n174 = Build Cluster Array(w469) -> (w467:cluster{dbl[]}[])
              n175 = Build Cluster Array(w468) -> (w466:cluster{dbl[]}[])
            }
            n176 = Interleave 1D Arrays(w455, w454) -> (w450:cluster{dbl[]}[])
            n177 = Interleave 1D Arrays(w453, w452) -> (w451:string[])
          }
        }
        n178 = Build Array (concatenate)(w446, w440) -> (w443:cluster{"Y  Array":dbl[]}[])
        n179 = Build Array (concatenate)(w445, w439) -> (w444:string[])
        n180 = Bundle By Name(cluster=w438, "data.Data"=w443, "data.wavenames"=w444) -> (w437:T12)
        n181 = call <vilib>:"Add State(s) to Queue__jki_lib_state_machine.vi"("State(s) in (\"\")"=w449) -> ("States Out"=w448:string)  [unwired: 14 in]
      }
      frame "File: Save ITX" {
        n182 = Unbundle By Name(w477) -> ("file.path"=w470:path, "file.Experiment Folder"=w476:string, "file.device"=w474:string, "file.Comments"=w473:string, "data.Data"=w472:cluster{"Y  Array":dbl[]}[], "data.wavenames"=w471:string[])
        n183 = Build Path(base path=w470, name or relative path=w476) -> (appended path=w475:path)
        n184 = call <userlib>:"LV to ITX XY2 AutoPlot.vi"("filename"=w474, "path"=w475, "Notes"=w473, "Data"=w472, "wavenames (.Vx, etc)"=w471) -> ()  [unwired: 10 in, 1 out]
        n185 = call <vilib>:"Add State(s) to Queue__jki_lib_state_machine.vi"("State(s) in (\"\")"=w480) -> ("States Out"=w479:string)  [unwired: 14 in]
      }
    }
  }
  "error out" <- w1
